vi "Build.vi"(9 "XYZTheta":dbl[](array[numeric]), 10 "Pattern Coordinates":dbl[][](array[numeric]), 11 "CAD Dispense in":refnum<class "CAD Dispense.lvclass">) -> (1 "Starting Coordinates":dbl[](array[numeric]), 3 "CAD Dispense out":refnum<class "CAD Dispense.lvclass">)   [LabVIEW 2019, in "CAD Dispense.lvclass"]
uses:
  CAD Dispense.lvclass
  CAD Dispense.lvclass/CAD Dispense.ctl
  <vilib>/Analysis/coordinate.llb/2D Cartesian Coordinate Rotation (Scalar).vi
  <vilib>/Analysis/NI_AALPro.lvlib
panel:
  out "array w/ subset deleted 2":T1(array[cluster])
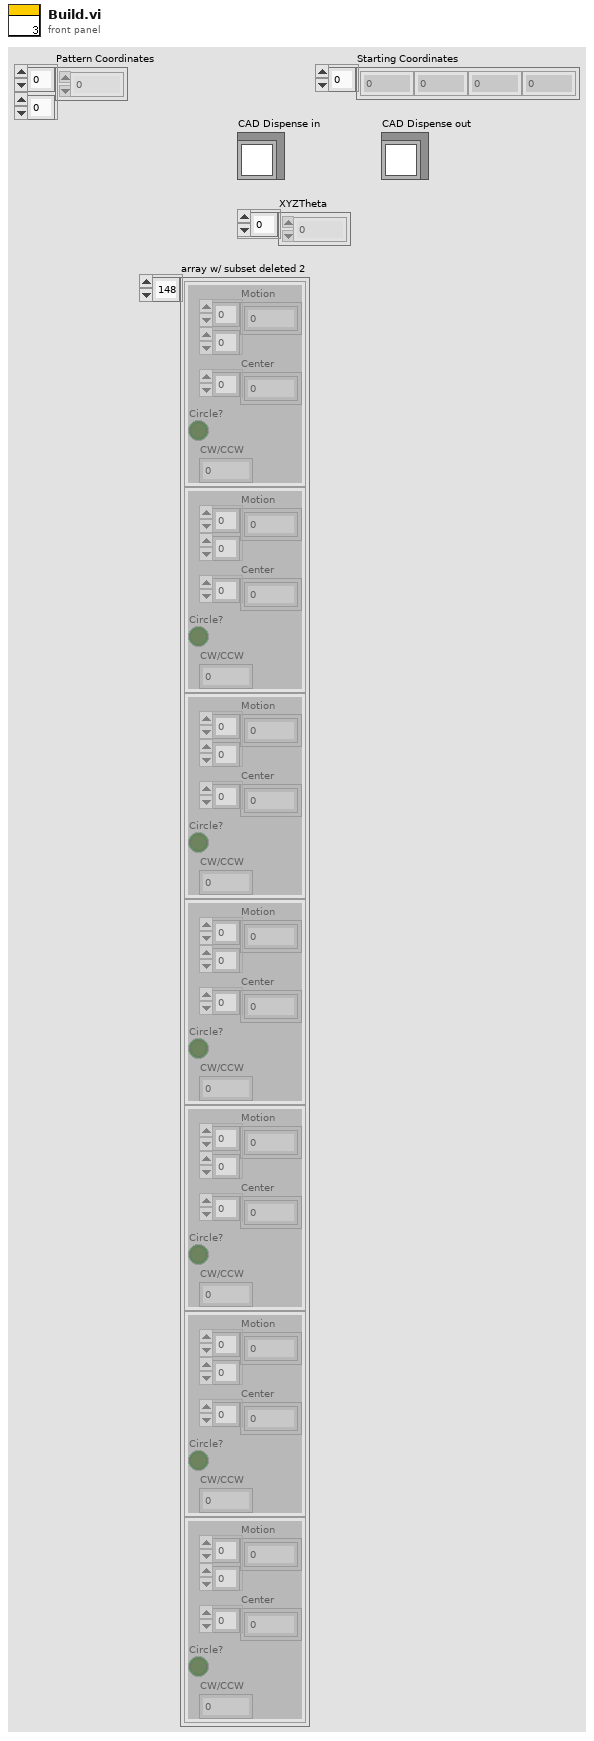
[diagram p1: front panel]
types:
  T1 = cluster{"Motion":dbl[][], "Center":dbl[], "Circle?":bool, "CW/CCW":dbl}[]
  T2 = cluster{"Motion":dbl[][], "Center":dbl[], "Circle?":bool, "CW/CCW":dbl}
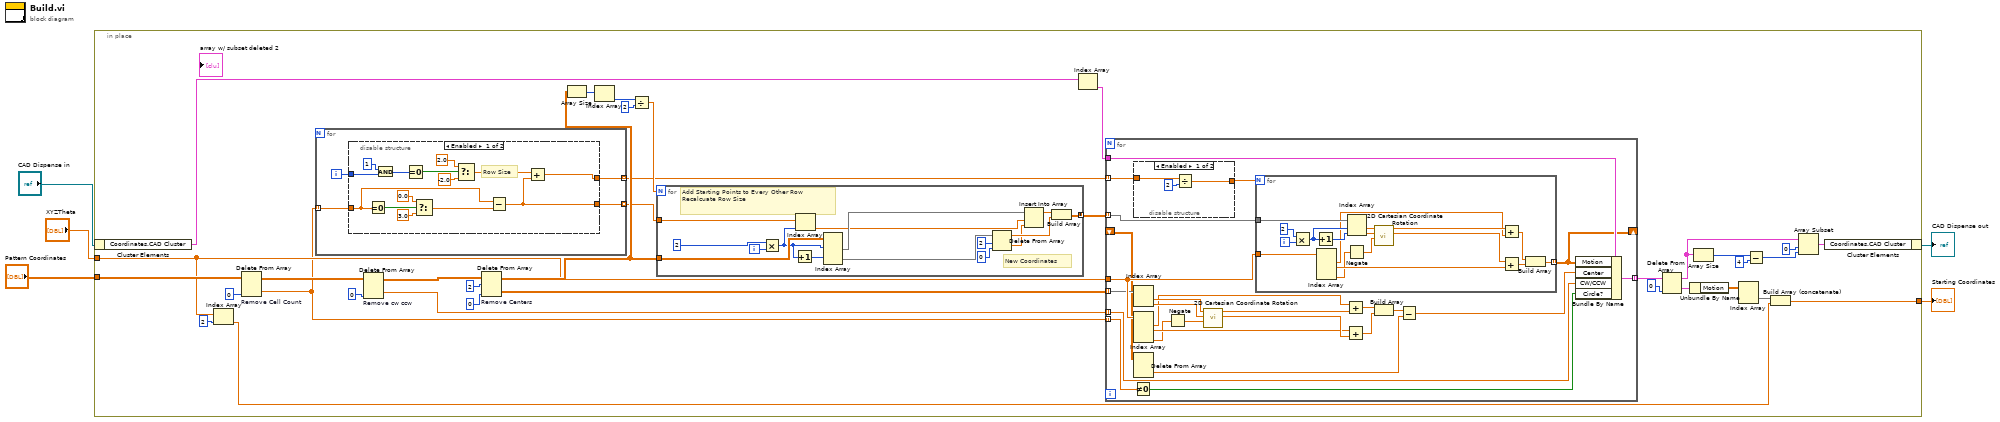
[diagram p0: block diagram]
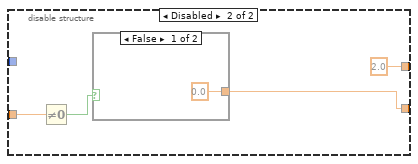
[diagram p2: hidden frame]
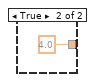
[diagram p3: hidden frame]
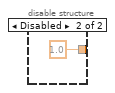
[diagram p4: hidden frame]
diagram:
  n1 = in-place {
    in-place-border: "XYZTheta" -> [w16]
    in-place-border: "Pattern Coordinates" -> [w27]
    in-place-border: [w13] -> w3
    n2 = in-place-cluster #1("CAD Dispense in") -> ("Coordinates.CAD Cluster"=w29:T1)
    n3 = Index Array(array=w16, index=2) -> (element=w14:dbl)
    n4 = Delete From Array "Remove Cell Count"(array=w27, index (col)=0 ("disabled index (col)")) -> (deleted portion=w6:dbl[], array with subset deleted=w34:dbl[][])  [unwired: 2 in]
    n5 = for {
      tunnel: w6 -> [w44] mode=indexing
      tunnel: [w43] -> w23 mode=indexing
      tunnel: [w42] -> w22 mode=indexing
      i -> [w41]
      n6 = disable-structure shown="Enabled" {
        disable-tunnel: w44 -> [w54 w61]
        disable-tunnel: w41 -> [w47 _]
        disable-tunnel: [w46 2.0] -> w43
        disable-tunnel: [w45 w59] -> w42
        frame Enabled {
          # "Row Size"
          n7 = Equal To 0?(x=w54) -> (x = 0?=w55:bool)
          n8 = And(x=1, y=w47) -> (x .and. y?=w50:i32)
          n9 = Equal To 0?(x=w50) -> (x = 0?=w48:bool)
          n10 = Select(t=0.0, s=w55, f=3.0) -> (s? t:f=w58:dbl)
          n11 = Select(t=2.0, s=w48, f=-2.0) -> (s? t:f=w51:dbl)
          n12 = Subtract(x=w54, y=w58) -> (x-y=w45:dbl)
          n13 = Add(x=w51, y=w45) -> (x+y=w46:dbl)
        }
        frame Disabled {
          n14 = Not Equal To 0?(x=w61) -> (x != 0?=w60:bool)
          n15 = case shown="False" w60 {
            tunnel: [0.0 4.0] -> w59
            frame False {
            }
            frame True {
            }
          }
        }
      }
    }
    n16 = Delete From Array "Remove cw ccw"(array=w34, index (col)=0 ("disabled index (col)")) -> (deleted portion=w39:dbl[], array with subset deleted=w35:dbl[][])  [unwired: 2 in]
    n17 = Delete From Array "Remove Centers"(array=w35, length=2, index (col)=0 ("disabled index (col)")) -> (deleted portion=w40:dbl[][], array with subset deleted=w36:dbl[][])  [unwired: 1 in]
    n18 = Array Size(array=w36) -> (size(s)=w37:i32[])
    n19 = Index Array(array=w37) -> (element=w26:i32)  [unwired: 1 in]
    n20 = Divide(x=w26, y=2) -> (x/y=w24:dbl)
    n21 = for {
      N: w24 -> [_]
      tunnel: w36 -> [w125]
      tunnel: [w117] -> w38 mode=concatenating
      tunnel: w22 -> [w112]
      i -> [w118]
      # "New Coordinates"
      # "Add Starting Points to Every Other Row\nRecalcuate Row Size"
      n22 = Multiply(x=2, y=w118) -> (x*y=w111:i32)
      n23 = Increment(x=w111) -> (x+1=w113:i32)
      n24 = Index Array(array=w112, index=w111) -> (element=w114:dbl)
      n25 = Index Array(array=w125, index (row) #1=w111, index (row) #2=w113) -> (element #1=w121:dbl[], element #2=w123:dbl[])  [unwired: 2 in]
      n26 = Delete From Array(array=w123, length=2, index=0) -> (deleted portion=w115:dbl[], array with subset deleted=w119:dbl[])
      n27 = Insert Into Array(array=w121, index=w114, new element=w115) -> (w120:dbl[])
      n28 = Build Array(w120, w119) -> (w117:dbl[][])
    }
    n29 = Index Array(array=w29) -> (element=w28:T2)  [unwired: 1 in]
    n30 = for {
      tunnel: w23 -> [w88] mode=indexing
      tunnel: w38 -> [w83] mode=indexing
      tunnel: w39 -> [w86] mode=indexing
      tunnel: w40 -> [w82] mode=indexing
      tunnel: w16 -> [w89]
      tunnel: w28 -> [w87]
      tunnel: [w84] -> w19 mode=indexing
      shift-right: [w72] -> _
      shift-left: _ -> [w70]
      tunnel: w6 -> [w65] mode=indexing
      n31 = Not Equal To 0?(x=w65) -> (x != 0?=w85:bool)
      n32 = disable-structure shown="Enabled" {
        disable-tunnel: w88 -> [w91 _]
        disable-tunnel: [w90 1.0] -> w79
        frame Enabled {
          n33 = Divide(x=w91, y=2) -> (x/y=w90:dbl)
        }
        frame Disabled {
        }
      }
      n34 = Index Array(array=w82) -> (element #1=w81:dbl, element #2=w80:dbl)  [unwired: 2 in]
      n35 = Index Array(array=w89) -> (element #1=w78:dbl, element #2=w73:dbl, element #4=w67:dbl)  [unwired: 4 in, 1 out]
      n36 = Delete From Array(array=w70) -> (deleted portion=w69:dbl[])  [unwired: 3 in, 1 out]
      n37 = Negate(x=w67) -> (-x=w66:dbl)
      n38 = call-poly <vilib>:"2D Cartesian Coordinate Rotation.vi"("theta"=w66, "y"=w80, "x"=w81) -> ("y out"=w75:dbl, "x out"=w77:dbl)  [unwired: 6 in, 1 out]
      n39 = for {
        N: w79 -> [_]
        tunnel: w83 -> [w110]
        tunnel: [w96] -> w72 mode=indexing
        tunnel: w89 -> [w106]
        i -> [w97]
        n40 = Multiply(x=2, y=w97) -> (x*y=w108:i32)
        n41 = Increment(x=w108) -> (x+1=w107:i32)
        n42 = Index Array(array=w106) -> (element #1=w99:dbl, element #2=w98:dbl, element #4=w95:dbl)  [unwired: 4 in, 1 out]
        n43 = Negate(x=w95) -> (-x=w94:dbl)
        n44 = Index Array(array=w110, index #1=w108, index #2=w107) -> (element #1=w102:dbl, element #2=w101:dbl)
        n45 = call-poly <vilib>:"2D Cartesian Coordinate Rotation.vi"("theta"=w94, "y"=w101, "x"=w102) -> ("y out"=w105:dbl, "x out"=w100:dbl)  [unwired: 6 in, 1 out]
        n46 = Add(x=w100, y=w99) -> (x+y=w104:dbl)
        n47 = Add(x=w105, y=w98) -> (x+y=w103:dbl)
        n48 = Build Array(w104, w103) -> (w96:dbl[])
      }
      n49 = Add(x=w78, y=w77) -> (x+y=w76:dbl)
      n50 = Add(x=w73, y=w75) -> (x+y=w74:dbl)
      n51 = Build Array(w76, w74) -> (w71:dbl[])
      n52 = Subtract(x=w71, y=w69) -> (x-y=w68:dbl[])
      n53 = Bundle By Name(cluster=w87, "Motion"=w72, "Center"=w68, "CW/CCW"=w86, "Circle?"=w85) -> (w84:T2)
    }
    n54 = Delete From Array(array=w19, index=0) -> (deleted portion=w21:T2, array with subset deleted=w12:T1)  [unwired: 1 in]
    n55 = Unbundle By Name(w21) -> ("Motion"=w18:dbl[][])
    n56 = Array Size(array=w12) -> (size(s)=w10:i32)
    n57 = Index Array(array=w18) -> (element=w17:dbl[])  [unwired: 2 in]
    n58 = Subtract(x=w10, y=4) -> (x-y=w8:i32)
    n59 = Build Array (concatenate)(w17, w14) -> (w13:dbl[])
    n60 = Array Subset(array=w12, index=0, length=w8) -> (w7:T1)
    n61 = in-place-cluster #1("Coordinates.CAD Cluster"=w7) -> (→"CAD Dispense out":refnum<class "CAD Dispense.lvclass">)
  }
  "Starting Coordinates" <- w3
